vi "Analyze Frequency Data.vi"(8 "error in":errorcluster, 11 "PAS in":refnum<class "PAS.lvclass">) -> (0 "error out":errorcluster, 1 "CellCharOut":T1(array[cluster]), 3 "PAS out":refnum<class "PAS.lvclass">)   [LabVIEW 2015, in "PAS.lvclass"]
uses:
  PAS.lvclass
  PAS.lvclass/PAS.ctl
  <vilib>/Analysis/4window.llb/windowTd.ctl
  <vilib>/measure/maspectr.llb/FFT Power Spectrum for 1 Chan.vi
  <vilib>/Analysis/NI_AALPro.lvlib
  <vilib>/measure/NI_MAPro.lvlib
  Data/Cell/PAS Cell Data.lvclass
  Data/Main/PAS Data.lvclass
  Cell/PAS Cell.lvclass
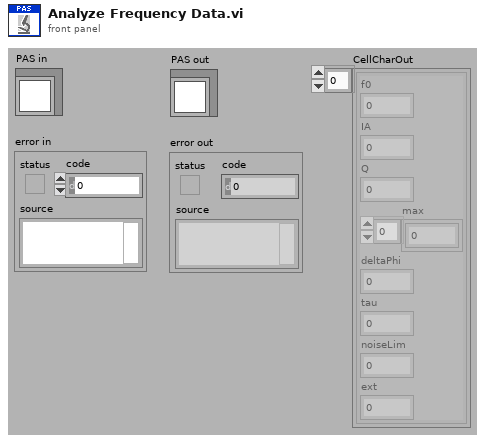
[diagram p1: front panel]
types:
  T1 = cluster{"f0":sgl, "IA":sgl, "Q":sgl, "max":dbl[], "deltaPhi":dbl, "tau":dbl, "noiseLim":dbl, "ext":dbl}[]
  T2 = typedef "NI_AALPro.lvlib/windowTd.ctl" = u32
  T3 = cluster{"f0":sgl, "IA":sgl, "Q":sgl, "max":dbl[], "deltaPhi":dbl, "tau":dbl, "noiseLim":dbl, "ext":dbl}
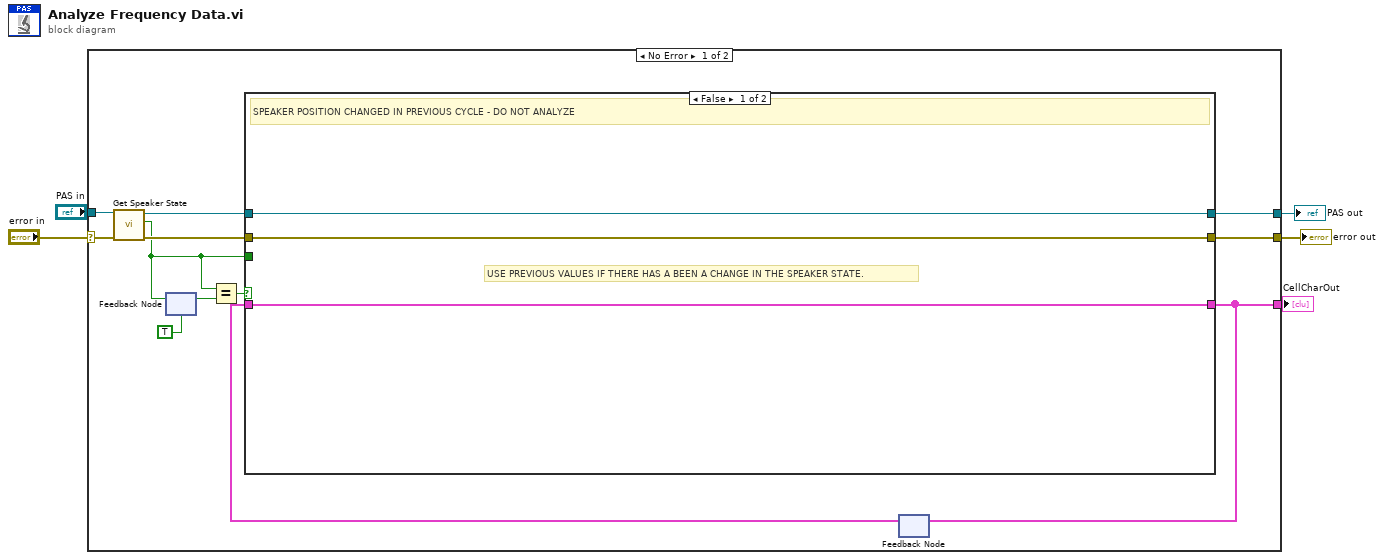
[diagram p0: block diagram]
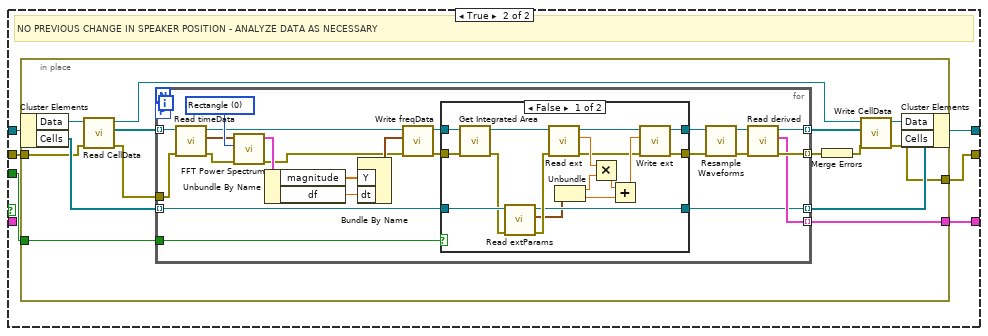
[diagram p2: hidden frame]
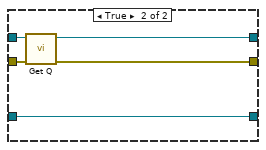
[diagram p3: hidden frame]
diagram:
  n1 = case shown="No Error" "error in" {
    selector: "error in" -> [w12 w87]
    tunnel: [w16 w87] -> w4
    tunnel: [w17 w86] -> w2
    tunnel: "PAS in" -> [w15 w86]
    tunnel: [w7 _] -> w1
    frame No Error {
      n2 = call "Get Speaker State.vi"("error in"=w12, "PAS in"=w15) -> ("error out"=w13:errorcluster, "State"=w9:bool, "PAS out"=w14:refnum<class "PAS.lvclass">)  [unwired: 7 in]
      n3 = feedback-in #1(w9) -> ()
      n4 = feedback #1(TRUE ("State")) -> (w10:bool)
      n5 = Equal?(x=w9, y=w10) -> (x = y?=w8:bool)
      n6 = feedback #2() -> (w6:T1)  [unwired: 1 in]
      n7 = case shown="False" w8 {
        tunnel: [w18 w26] -> w7
        tunnel: [w19 w25] -> w17
        tunnel: [w20 w24] -> w16
        tunnel: w14 -> [w19 w23]
        tunnel: w13 -> [w20 w22]
        tunnel: w9 -> [_ w21]
        tunnel: w6 -> [w18 _]
        frame False {
          # "USE PREVIOUS VALUES IF THERE HAS A BEEN A CHANGE IN THE SPEAKER STATE."
          # "SPEAKER POSITION CHANGED IN PREVIOUS CYCLE - DO NOT ANALYZE"
        }
        frame True {
          # "NO PREVIOUS CHANGE IN SPEAKER POSITION - ANALYZE DATA AS NECESSARY"
          n8 = in-place {
            in-place-border: [w32] -> w24
            in-place-border: [w37] -> w26
            in-place-border: w22 -> [w28]
            in-place-border: w21 -> [w30]
            n9 = in-place-cluster #3(w23) -> ("Data"=w29:refnum<class "PAS Data.lvclass">, "Cells"=w36:refnum<class "PAS Cell.lvclass">[])
            n10 = call "Read CellData.vi"("error in"=w28, "PAS Data in"=w29) -> ("error out"=w27:errorcluster, "CellData"=w39:refnum<class "PAS Cell Data.lvclass">[], "PAS Data out"=w38:refnum<class "PAS Data.lvclass">)  [unwired: 7 in]
            n11 = for {
              tunnel: w39 -> [w52] mode=indexing
              tunnel: w27 -> [w51]
              tunnel: [w48] -> w40 mode=indexing
              tunnel: [w47] -> w34 mode=indexing
              workers-P: _ -> [_]
              tunnel: w30 -> [w45]
              tunnel: [w46] -> w37 mode=indexing
              tunnel: w36 -> [w42] mode=indexing
              tunnel: [w41] -> w35 mode=indexing
              w61 = T2 0 items=["Rectangle"=0, "Hanning"=1, "Hamming"=2, "Blackman-Harris"=3, "Exact Blackman"=4, "Blackman"=5, "Flat Top"=6, "4 Term B-Harris "=7, "7 Term B-Harris"=8, "Low Sidelobe"=9, "Blackman Nuttall"=11, "Triangle"=30, "Bartlett-Hanning"=31, "Bohman"=32, "Parzen"=33, "Welch"=34, "Kaiser"=60, "Dolph-Chebyshev"=61, "Gaussian"=62] ("window")
              n12 = call "Read timeData.vi"("error in"=w51, "PAS Cell Data in"=w52) -> ("error out"=w56:errorcluster, "timeData"=w59:waveform(i16), "PAS Cell Data out"=w57:refnum<class "PAS Cell Data.lvclass">)  [unwired: 7 in]
              n13 = call-poly <vilib>:"FFT Power Spectrum.vi"("error in (no error)"=w56, "window"=w61, "time signal"=w59) -> ("error out"=w55:errorcluster, "power spectrum"=w60:cluster{"f0":dbl, "df":dbl, "magnitude":dbl[]})  [unwired: 3 in, 4 out]
              n14 = Unbundle By Name(w60) -> ("magnitude"=w63:dbl[], "df"=w62:dbl)
              n15 = Bundle By Name("Y"=w63, "dt"=w62) -> (w58:waveform(dbl))  [unwired: 1 out]
              n16 = call "Write freqData.vi"("error in (no error)"=w55, "freqData"=w58, "PAS Cell Data in"=w57) -> ("error out"=w53:errorcluster, "PAS Cell Data out"=w54:refnum<class "PAS Cell Data.lvclass">)  [unwired: 7 in]
              n17 = case shown="False" w45 {
                tunnel: w54 -> [w80 w85]
                tunnel: w53 -> [w79 w84]
                tunnel: [w65 w83] -> w49
                tunnel: [w64 w82] -> w50
                tunnel: w42 -> [w78 w81]
                tunnel: [w74 w81] -> w41
                frame False {
                  n18 = call "Get Integrated Area.vi"("error in"=w79, "PAS Cell Data in"=w80) -> ("error out"=w77:errorcluster, "PAS Cell Data out"=w76:refnum<class "PAS Cell Data.lvclass">)  [unwired: 8 in]
                  n19 = call "Read extParams.vi"("error in"=w77, "PAS Cell in"=w78) -> ("error out"=w75:errorcluster, "extParams"=w73:cluster{"slope":sgl, "zero":sgl}, "PAS Cell out"=w74:refnum<class "PAS Cell.lvclass">)  [unwired: 7 in]
                  n20 = call "Read ext.vi"("error in"=w75, "PAS Cell Data in"=w76) -> ("error out"=w66:errorcluster, "ext"=w71:dbl, "PAS Cell Data out"=w72:refnum<class "PAS Cell Data.lvclass">)  [unwired: 7 in]
                  n21 = Unbundle(w73) -> ("slope"=w70:sgl, "zero"=w68:sgl)
                  n22 = Multiply(x=w71, y=w70) -> (x*y=w69:dbl)
                  n23 = Add(x=w69, y=w68) -> (x+y=w67:dbl)
                  n24 = call "Write ext.vi"("error in"=w66, "ext"=w67, "PAS Cell Data in"=w72) -> ("error out"=w65:errorcluster, "PAS Cell Data out"=w64:refnum<class "PAS Cell Data.lvclass">)  [unwired: 7 in]
                }
                frame True {
                  n25 = call "Get Q.vi"("error in"=w84, "PAS Cell Data in"=w85) -> ("error out"=w83:errorcluster, "PAS Cell Data out"=w82:refnum<class "PAS Cell Data.lvclass">)  [unwired: 8 in]
                }
              }
              n26 = call "Resample Waveforms.vi"("error in"=w49, "PAS Cell Data in"=w50) -> ("error out"=w44:errorcluster, "PAS Cell Data out"=w43:refnum<class "PAS Cell Data.lvclass">)  [unwired: 8 in]
              n27 = call "Read derived.vi"("error in"=w44, "PAS Cell Data in"=w43) -> ("error out"=w47:errorcluster, "derived"=w46:T3, "PAS Cell Data out"=w48:refnum<class "PAS Cell Data.lvclass">)  [unwired: 7 in]
            }
            n28 = Merge Errors(w34) -> (w33:errorcluster)
            n29 = call "Write CellData.vi"("error in"=w33, "CellData"=w40, "PAS Data in"=w38) -> ("error out"=w32:errorcluster, "PAS Data out"=w31:refnum<class "PAS Data.lvclass">)  [unwired: 7 in]
            n30 = in-place-cluster #3("Data"=w31, "Cells"=w35) -> (w25:refnum<class "PAS.lvclass">)
          }
        }
      }
      n31 = feedback-in #2(w7) -> ()
    }
    frame Error {
    }
  }
  "error out" <- w4
  "PAS out" <- w2
  "CellCharOut" <- w1
